vi "Import from CSV.vi"(8 "error in":errorcluster, 11 "Engine in":refnum<class "Engine.lvclass">) -> (0 "error out":errorcluster, 2 "VI Information Array":T1[](array[typedef]), 3 "Engine out":refnum<class "Engine.lvclass">)   [LabVIEW 2017, in "Engine.lvclass"]
uses:
  Engine.lvclass
  VI Information.ctl
  Engine.lvclass/Engine.ctl
  <vilib>/Utility/file.llb/Read Delimited Spreadsheet (string).vi
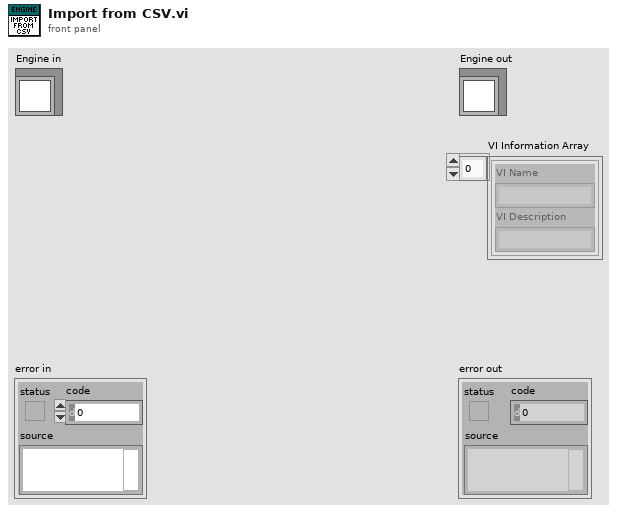
[diagram p1: front panel]
types:
  T1 = typedef "Engine.lvclass/VI Information.ctl" = cluster{"VI Name":string, "VI Description":string}
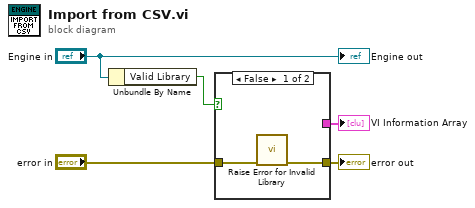
[diagram p0: block diagram]
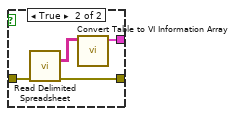
[diagram p2: hidden frame]
diagram:
  n1 = Unbundle By Name("Engine in") -> ("Valid Library"=w2:bool)
  n2 = case shown="False" w2 {
    tunnel: [w6 w11] -> w5
    tunnel: "error in" -> [w7 w10]
    tunnel: [_ w9] -> w1
    frame False {
      n3 = call "Raise Error for Invalid Library.vi"("error in"=w7) -> ("error out"=w6:errorcluster)  [unwired: 10 in]
    }
    frame True {
      n4 = call-poly <vilib>:"Read Delimited Spreadsheet.vi"("error in (no error)"=w10) -> ("all rows"=w8:string[][], "error out"=w11:errorcluster)  [unwired: 9 in, 4 out]
      n5 = call "Convert Table to VI Information Array.vi"("Array Out"=w8) -> ("VI Information Array"=w9:T1[])  [unwired: 10 in]
    }
  }
  "error out" <- w5
  "VI Information Array" <- w1
  "Engine out" <- "Engine in"
